vi "Set Default Column Headers.vi"(8 "error in (no error)":errorcluster, 11 "ResultTree in":refnum<class "Result Tree.lvclass">) -> (0 "error out":errorcluster, 3 "ResultTree out":refnum<class "Result Tree.lvclass">)   [LabVIEW 2017, in "Result Tree.lvclass"]
doc: "Sets the default column headers."
uses:
  Result Tree.lvclass
  Result Tree.lvclass/Result Tree.ctl
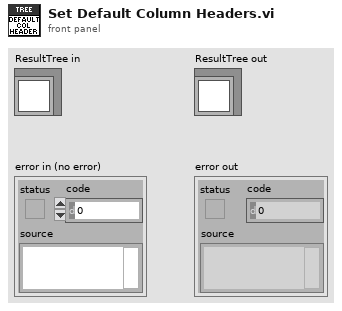
[diagram p1: front panel]
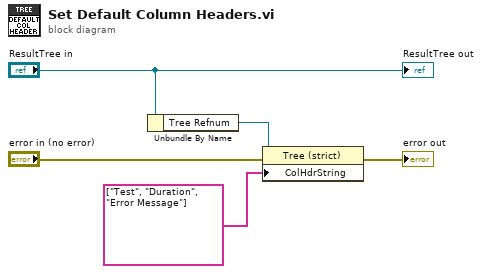
[diagram p0: block diagram]
diagram:
  n1 = Unbundle By Name("ResultTree in") -> ("Tree Refnum"=w2:refnum<vi>)
  n2 = property class="Tree (strict)"(reference=w2, error in="error in (no error)", "ColHdrString"=string[] ["Test", "Duration", "Error Message"] ("Column Header Strings[]")) -> (error out=→"error out":errorcluster)  [unwired: 1 out]
  "ResultTree out" <- "ResultTree in"
